vi "get mappable tags.vi"(11 "engine configuration in":refnum<class "engine configuration.lvclass">) -> (1 "Output Tags":string[](array[string]), 2 "Process Variable Tags":string[](array[string]), 3 "Setpoint Tags":string[](array[string]))   [LabVIEW 2013]
uses:
  <vilib>/NI/Module Execution Interface/Engine Configuration/engine configuration.lvclass
  PID array element.ctl
  <vilib>/NI/Tag Bus/tag/tag descriptor.lvclass/tag descriptor.ctl
  <vilib>/NI/Tag Bus/tag/read tag name.vi
  module/configuration/PID Module configuration.lvclass
  <vilib>/NI/Tag Bus/tag/tag descriptor.lvclass
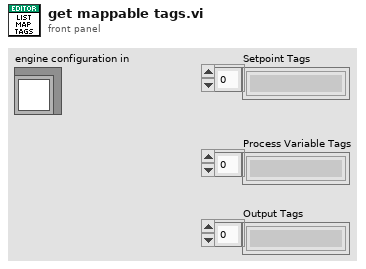
[diagram p1: front panel]
types:
  T1 = typedef "PID Module configuration.lvclass/PID array element.ctl" = cluster{"Loop ID":string, "Tags":cluster{"Setpoint":string, "Process Variable":string, "Output":string}, "Gains":cluster{"P":dbl, "I":dbl, "D":dbl}, "Range":cluster{"High":dbl, "Low":dbl}}
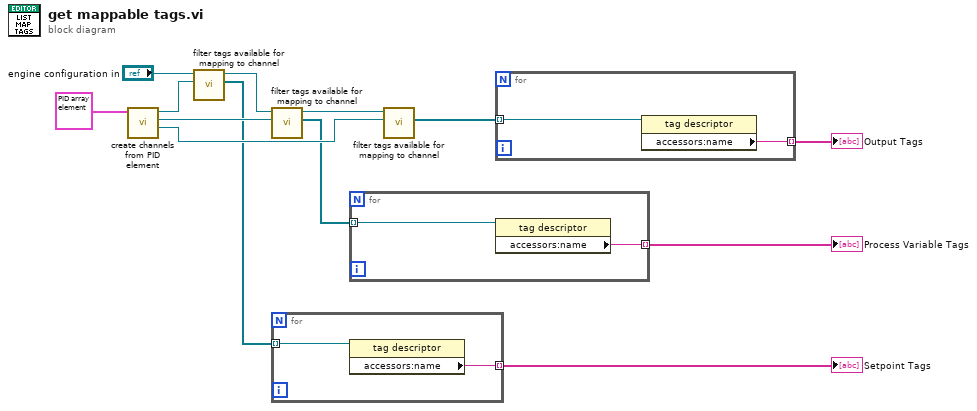
[diagram p0: block diagram]
diagram:
  n1 = call "create channels from PID element.vi"("line item in"=T1 {"Loop ID"="", "Tags"={"Setpoint"="", "Process Variable"="", "Output"=""}, "Gains"={"P"=0.0, "I"=0.0, "D"=0.0}, "Range"={"High"=0.0, "Low"=0.0}}) -> ("Output Channel Out"=w11:refnum<class "TBM channel.lvclass">, "Process Variable Channel Out"=w6:refnum<class "TBM channel.lvclass">, "Setpoint Channel Out"=w2:refnum<class "TBM channel.lvclass">)  [unwired: 8 in]
  n2 = call <vilib>:"filter tags available for mapping to channel.vi"("channel to map to"=w2, "engine configuration in"="engine configuration in") -> ("filtered tags"=w3:refnum<class "tag descriptor.lvclass">[], "engine configuration out"=w1:refnum<class "engine configuration.lvclass">)  [unwired: 8 in]
  n3 = call <vilib>:"filter tags available for mapping to channel.vi"("channel to map to"=w6, "engine configuration in"=w1) -> ("filtered tags"=w8:refnum<class "tag descriptor.lvclass">[], "engine configuration out"=w10:refnum<class "engine configuration.lvclass">)  [unwired: 8 in]
  n4 = for {
    tunnel: w3 -> [w15] mode=indexing
    tunnel: [w14] -> w4 mode=indexing
    n5 = property class="tag descriptor"(reference=w15) -> ("accessors:name"=w14:string)  [unwired: 1 in, 2 out]
  }
  "Setpoint Tags" <- w4
  n6 = for {
    tunnel: w8 -> [w17] mode=indexing
    tunnel: [w16] -> w9 mode=indexing
    n7 = property class="tag descriptor"(reference=w17) -> ("accessors:name"=w16:string)  [unwired: 1 in, 2 out]
  }
  "Process Variable Tags" <- w9
  n8 = call <vilib>:"filter tags available for mapping to channel.vi"("channel to map to"=w11, "engine configuration in"=w10) -> ("filtered tags"=w12:refnum<class "tag descriptor.lvclass">[])  [unwired: 8 in, 1 out]
  n9 = for {
    tunnel: w12 -> [w19] mode=indexing
    tunnel: [w18] -> w13 mode=indexing
    n10 = property class="tag descriptor"(reference=w19) -> ("accessors:name"=w18:string)  [unwired: 1 in, 2 out]
  }
  "Output Tags" <- w13
